vi "SineOrSawtooth2.vi"(7 "Sine\nSawtooth":bool, 8 "error in (no error)":errorcluster, 9 "Amplitude":dbl[unit], 10 "2*pi*f":dbl[unit], 11 "Time":dbl[](array[numeric])) -> (0 "error out":errorcluster, 3 "Signal":dbl[](array[numeric]))   [LabVIEW 2010]
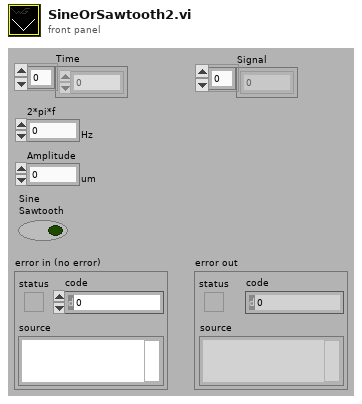
[diagram p1: front panel]
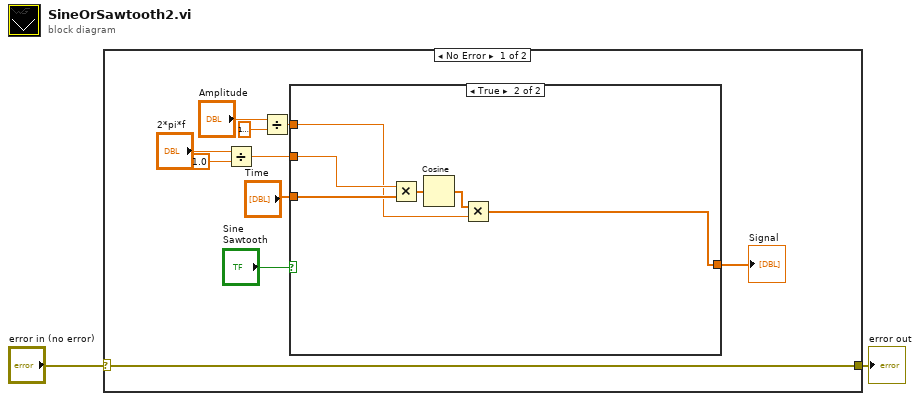
[diagram p0: block diagram]
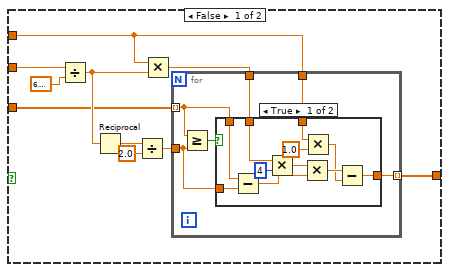
[diagram p2: hidden frame]
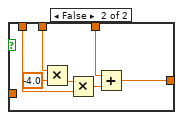
[diagram p3: hidden frame]
diagram:
  n1 = case shown="No Error" "error in (no error)" {
    selector: "error in (no error)" -> [w12 w53]
    tunnel: [w12 w53] -> w1
    frame No Error {
      n2 = Divide(x="2*pi*f", y=dbl[unit] 1.0 ("x")) -> (x/y=w8:dbl)
      n3 = Divide(x="Amplitude", y=dbl[unit] 1e-06) -> (x/y=w9:dbl)
      n4 = case shown="True" "Sine\nSawtooth" {
        tunnel: w9 -> [w21 w48]
        tunnel: w8 -> [w19 w50]
        tunnel: "Time" -> [w14 w49]
        tunnel: [w13 w47] -> w11
        frame False {
          n5 = Divide(x=w19, y=6.283185307179586) -> (x/y=w15:dbl)
          n6 = Reciprocal(x=w15) -> (1/x=w18:dbl)
          n7 = Divide(x=w18, y=2.0) -> (x/y=w16:dbl)
          n8 = Multiply(x=w21, y=w15) -> (x*y=w22:dbl)
          n9 = for {
            tunnel: w22 -> [w25]
            tunnel: w14 -> [w24] mode=indexing
            tunnel: w21 -> [w27]
            tunnel: w16 -> [w23]
            tunnel: [w26] -> w13 mode=indexing
            n10 = Greater Or Equal?(x=w24, y=w23) -> (x >= y?=w28:bool)
            n11 = case shown="True" w28 {
              tunnel: w24 -> [w29 w40]
              tunnel: w27 -> [w32 w43]
              tunnel: [w35 w42] -> w26
              tunnel: w25 -> [w37 w41]
              tunnel: w23 -> [w31 _]
              frame True {
                n12 = Subtract(x=w29, y=w31) -> (x-y=w30:dbl)
                n13 = Multiply(x=w37, y=4) -> (x*y=w39:dbl)
                n14 = Multiply(x=w39, y=w30) -> (x*y=w36:dbl)
                n15 = Multiply(x=w32, y=1.0) -> (x*y=w33:dbl)
                n16 = Subtract(x=w36, y=w33) -> (x-y=w35:dbl)
              }
              frame False {
                n17 = Multiply(x=w41, y=-4.0) -> (x*y=w46:dbl)
                n18 = Multiply(x=w46, y=w40) -> (x*y=w45:dbl)
                n19 = Add(x=w43, y=w45) -> (x+y=w42:dbl)
              }
            }
          }
        }
        frame True {
          n20 = Multiply(x=w50, y=w49) -> (x*y=w52:dbl[])
          n21 = Cosine(x=w52) -> (cos(x)=w51:dbl[])
          n22 = Multiply(x=w51, y=w48) -> (x*y=w47:dbl[])
        }
      }
      "Signal" <- w11
    }
    frame Error {
    }
  }
  "error out" <- w1
